vi "Get Property - Include Direction Section.vi"(8 "error in":errorcluster, 11 "custom device":u64) -> (0 "error out":errorcluster, 3 "Value":bool)   [LabVIEW 2020, in "AIM MIL-STD-1553 Scripting.lvlib"]
uses:
  AIM MIL-STD-1553 Scripting.lvlib
  Constants.vi
  <vilib>/NI VeriStand/Custom Device API/Get Item Property (Boolean).vi
  <vilib>/NI VeriStand/Custom Device API/Custom Device API.lvlib
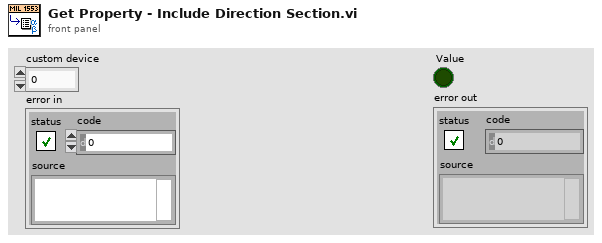
[diagram p1: front panel]
types:
  T1 = typedef "Custom Device API.lvlib/Custom Device Item Ref.ctl" = u64
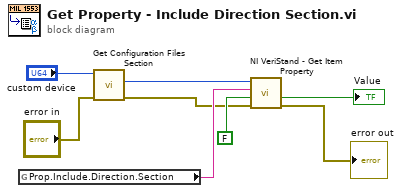
[diagram p0: block diagram]
diagram:
  n1 = global read "Constants.vi" "Prop.Include.Direction.Section"() -> (w8:string)
  n2 = call "Get Configuration Files Section.vi"("error in"="error in", "custom device"="custom device") -> ("error out"=w3:errorcluster, "configuration files section"=w1:T1)  [unwired: 6 in, 2 out]
  n3 = call-poly <vilib>:"NI VeriStand - Get Item Property.vi"("error in (no error)"=w3, "Default Value"=FALSE, "Property Name"=w8, "Item Ref in"=w1) -> ("error out"=→"error out":errorcluster, "Value"=→"Value":bool)  [unwired: 4 in, 2 out]
